vi "0037-Sub_calc_SHT31.vi"(11 "Data":u8[](array[numeric])) -> (2 "数値":dbl, 3 "数値 2":dbl)   [LabVIEW 2014]
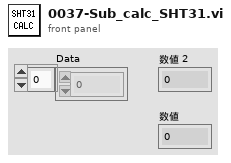
[diagram p1: front panel]
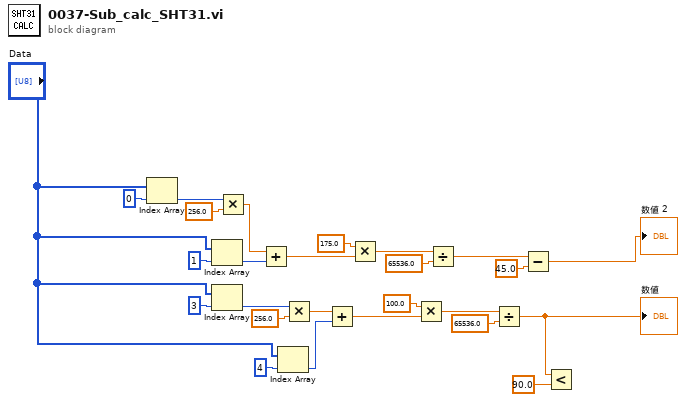
[diagram p0: block diagram]
diagram:
  n1 = Index Array(array="Data", index=0 ("指標")) -> (element=w3:u8)
  n2 = Index Array(array="Data", index=1 ("指標")) -> (element=w6:u8)
  n3 = Index Array(array="Data", index=3 ("指標")) -> (element=w21:u8)
  n4 = Multiply(x=w3, y=256.0) -> (x*y=w5:dbl)
  n5 = Add(x=w5, y=w6) -> (x+y=w8:dbl)
  n6 = Index Array(array="Data", index=4 ("指標")) -> (element=w22:u8)
  n7 = Multiply(x=w21, y=256.0) -> (x*y=w16:dbl)
  n8 = Add(x=w16, y=w22) -> (x+y=w18:dbl)
  n9 = Multiply(x=175.0, y=w8) -> (x*y=w9:dbl)
  n10 = Multiply(x=100.0, y=w18) -> (x*y=w19:dbl)
  n11 = Divide(x=w9, y=65536.0) -> (x/y=w11:dbl)
  n12 = Divide(x=w19, y=65536.0) -> (x/y=w24:dbl)
  "数値" <- w24
  n13 = Subtract(x=w11, y=45.0) -> (x-y=→"数値 2":dbl)
  n14 = Less?(x=w24, y=90.0) -> ()  [unwired: 1 out]
